vi "CSM Execute - Edit Script.vi"(6 "Mouse Position":T1, 8 "User VI Ref":refnum<vi>, 9 "Menu Item Tag Suffix":string, 10 "Remaining Items":refnum<vi>[](array[refnum]), 11 "Affected Items":T2) -> (0 "Fail transaction?":bool)   [LabVIEW 2017]
doc: "This VI is part of a plug-in for modifying the LabVIEW shortcut menus. This is the execute VI which is called when the shortcut menu is chosen by the user. It performs the action of the selected menu item."
uses:
  CSM Execute - Shortcut Menu Plug-In.ctl
  <vilib>/Utility/miscctls.llb/LVPositionTypeDef.ctl
  Communicable State Machine.lvlib
panel:
  # "All controls on this panel except \"Affected Items\" have been locked to prevent accidental edits. Changing the control names or types, other than the elements of the \"Affected Items\" cluster will make the VI unusable as a menu plugin.\n\nSee Context Help for each control for details about its use."
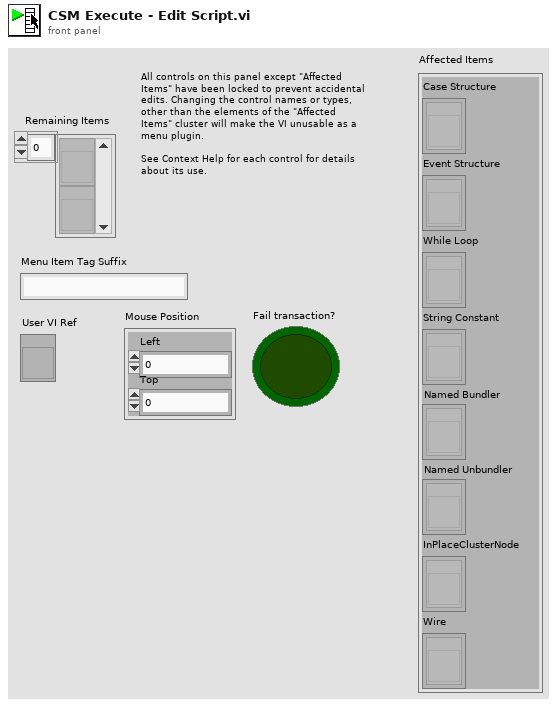
[diagram p1: front panel]
types:
  T1 = typedef "LVPositionTypeDef.ctl" = cluster{"Left":i32, "Top":i32}
  T2 = typedef "CSM Execute - Shortcut Menu Plug-In.ctl" = cluster{"Case Structure":refnum<vi>[], "Event Structure":refnum<vi>[], "While Loop":refnum<vi>[], "String Constant":refnum<vi>[], "Named Bundler":refnum<vi>[], "Named Unbundler":refnum<vi>[], "InPlaceClusterNode":refnum<vi>[], "Wire":refnum<vi>[]}
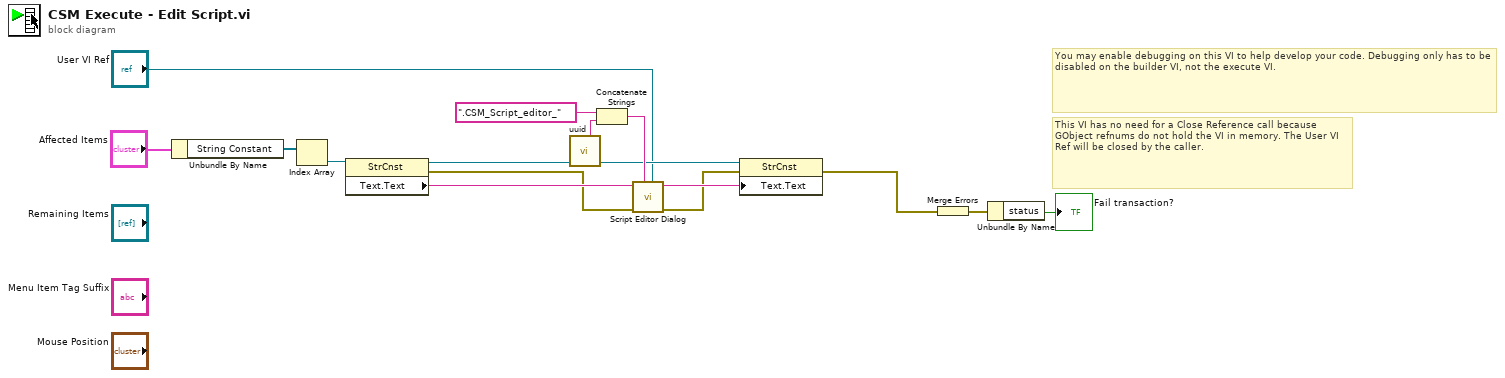
[diagram p0: block diagram]
diagram:
  # "You may enable debugging on this VI to help develop your code. Debugging only has to be disabled on the builder VI, not the execute VI."
  # "This VI has no need for a Close Reference call because GObject refnums do not hold the VI in memory. The User VI Ref will be closed by the caller."
  n1 = Unbundle By Name("Affected Items") -> ("String Constant"=w12:refnum<vi>[])
  n2 = Index Array(array=w12) -> (element=w11:refnum<vi>)  [unwired: 1 in]
  n3 = property class="StrCnst"(reference=w11) -> (reference out=w5:refnum<vi>, error out=w3:errorcluster, "Text.Text"=w10:string)  [unwired: 1 in]
  n4 = call "uuid.vi"() -> ("UUID"=w7:string)  [unwired: 11 in]
  n5 = Concatenate Strings(".CSM_Script_editor_" ("Name(\"\" to use uuid)"), w7) -> (w8:string)
  n6 = call "Script Editor Dialog.vi"("VI Refnum"="User VI Ref", "Name (\"\" to Use Uuid)"=w8, "Error In"=w3, "Script"=w10) -> ("Error Out"=w4:errorcluster, "Script Out"=w6:string)  [unwired: 6 in]
  n7 = property class="StrCnst"(reference=w5, error in=w4, "Text.Text"=w6) -> (error out=w2:errorcluster)  [unwired: 1 out]
  n8 = Merge Errors(w2) -> (w14:errorcluster)
  n9 = Unbundle By Name(w14) -> ("status"=→"Fail transaction?":bool)
